vi "move motor.vi"() -> ()   [LabVIEW 2013]
panel:
  out "steps performed":i32=1
  in  "direction":enum16{"counter-clockwise", "clockwise"}(ring)
  in  "steps":i32=1
  out "error out":errorcluster
  in  "error in (no error)":errorcluster
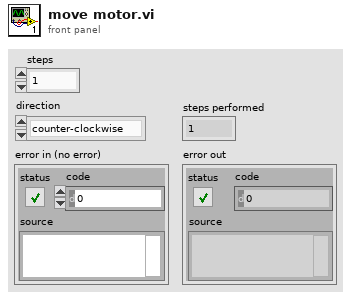
[diagram p1: front panel]
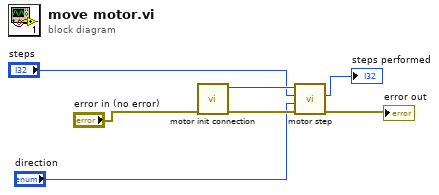
[diagram p0: block diagram]
diagram:
  n1 = call "motor init connection.vi"("error in (no error)"="error in (no error)") -> ("error out"=w5:errorcluster, "Handle Out"=w7:i32)  [unwired: 9 in]
  n2 = call "motor step.vi"("error in (no error)"=w5, "direction"="direction", "steps"="steps", "Handle In"=w7) -> ("error out"=→"error out":errorcluster, "steps performed"=→"steps performed":i32)  [unwired: 5 in, 1 out]
